vi "军蚁-初始化结果界面.vi"(8 "error in (no error)":errorcluster, 11 "基路径":path) -> (0 "error out":errorcluster, 1 "Fail":string, 2 "pass":string, 3 "Image Out":T1(plugin-control))   [LabVIEW 2017]
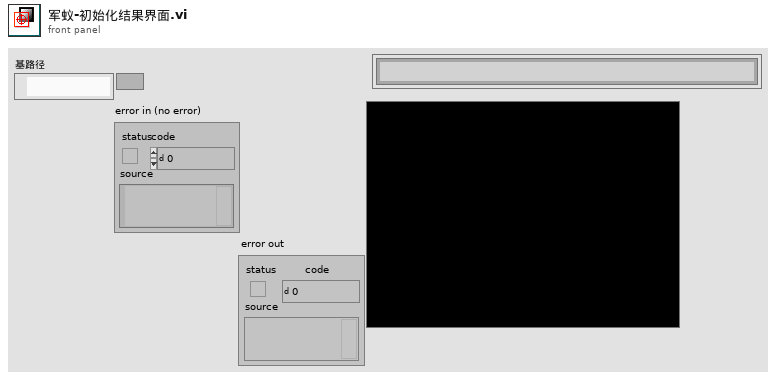
[diagram p1: front panel]
types:
  T1 = typedef "IMAQ Image.ctl" = refnum<image>
  T2 = cluster{"Cent X":dbl, "Cent Y":dbl, "Big1 R":dbl, "Small1 R":dbl, "Big2 R":dbl, "Small2 R":dbl, "Start_OutSide":dbl, "Start_InSide":dbl}
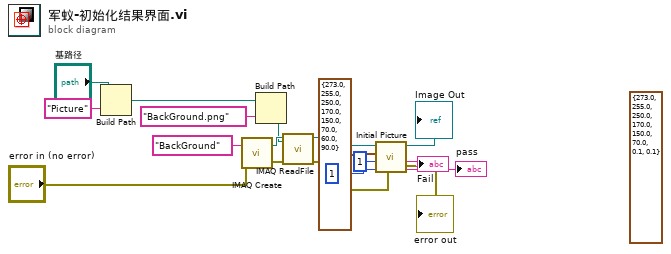
[diagram p0: block diagram]
diagram:
  (unwired) T2 {"Cent X"=273.0, "Cent Y"=255.0, "Big1 R"=250.0, "Small1 R"=170.0, "Big2 R"=150.0, "Small2 R"=70.0, "Start_OutSide"=0.1, "Start_InSide"=0.1} ("中心位置")
  n1 = Build Path(base path="基路径", name or relative path="Picture" ("名称或相对路径")) -> (appended path=w8:path)
  n2 = call "IMAQ Create"("Image Name"="BackGround", "error in (no error)"="error in (no error)") -> ("New Image"=w17:T1, "error out"=w16:errorcluster)  [unwired: 3 in]
  n3 = Build Path(base path=w8, name or relative path="BackGround.png" ("名称或相对路径")) -> (appended path=w6:path)
  n4 = call "IMAQ ReadFile"("File Path"=w6, "error in (no error)"=w16, "Image"=w17) -> ("error out"=w2:errorcluster, "Image Out"=w15:T1)  [unwired: 4 in, 3 out]
  n5 = call "Initial Picture.vi"("error in (no error)"=w2, "Pass"=1, "fail"=1, "中心位置"=T2 {"Cent X"=273.0, "Cent Y"=255.0, "Big1 R"=250.0, "Small1 R"=170.0, "Big2 R"=150.0, "Small2 R"=70.0, "Start_OutSide"=60.0, "Start_InSide"=90.0}, "Image In"=w15) -> ("pass"=→"pass":string, "fail"=→"Fail":string, "Image Out"=→"Image Out":T1, "error out"=→"error out":errorcluster)  [unwired: 3 in]
